vi "Test.vi"() -> ()   [LabVIEW 2009]
uses:
  LV-BME Interface/BME_DG_TriggerSettings.ctl
  LV-BME Interface/ChnlSettings.ctl
  LV-BME Interface/ChnlWithModulo.ctl
panel:
  out "Array":T1(array[cluster])=[{"Master"=TRUE, "DG_Product"=34, "SlotNumber"=5, "return code"=0}, {"Master"=FALSE, "DG_Product"=33, "SlotNumber"=7, "return code"=0}, {"Master"=FALSE, "DG_Product"=33, "SlotNumber"=9, "return code"=0}, {"Master"=FALSE, "DG_Product"=33, "SlotNumber"=11, "return code"=0}]
  in  "Chnl Settings T, A, B":T2[](array[typedef])=[{" Delay (µs)"=0.0, "TriggerModulo"=1, "On? (false)"=TRUE, "PositiveVoltage?(true)"=TRUE, "50OhmTerminated? "=FALSE, "25OhmOutput?"=FALSE}, {" Delay (µs)"=0.0, "TriggerModulo"=4, "On? (false)"=TRUE, "PositiveVoltage?(true)"=TRUE, "50OhmTerminated? "=FALSE, "25OhmOutput?"=FALSE}, {" Delay (µs)"=0.0, "TriggerModulo"=8, "On? (false)"=TRUE, "PositiveVoltage?(true)"=TRUE, "50OhmTerminated? "=TRUE, "25OhmOutput?"=FALSE}] {"TriggerModulo" min=1 max=1000000; "Delay (µs)" min=0.0 max=100000000.0 format="%.5f"}
  in  "Chnl Settings T, A, B written":T2[](array[typedef])=[{" Delay (µs)"=0.0, "TriggerModulo"=1, "On? (false)"=TRUE, "PositiveVoltage?(true)"=TRUE, "50OhmTerminated? "=FALSE, "25OhmOutput?"=FALSE}, {" Delay (µs)"=0.0, "TriggerModulo"=4, "On? (false)"=TRUE, "PositiveVoltage?(true)"=TRUE, "50OhmTerminated? "=FALSE, "25OhmOutput?"=FALSE}, {" Delay (µs)"=0.0, "TriggerModulo"=8, "On? (false)"=TRUE, "PositiveVoltage?(true)"=TRUE, "50OhmTerminated? "=TRUE, "25OhmOutput?"=FALSE}] {"TriggerModulo" min=1 max=1000000; "Delay (µs)" min=0.0 max=100000000.0 format="%.5f"}
  out "Update chnl errors":errorcluster[](array[cluster])
  in  "update chnl settings":bool=TRUE
  out "counters remain":u32[](array[numeric])=[1, 2, 6]
  out "activate":i32[](array[numeric])
  in  "Activate":bool=TRUE
  out "Chnl States":i32[][](array[numeric])
  in  "ReadStatus":bool=TRUE
  in  "stop 2":bool=TRUE
  in  "stop":bool=TRUE
  out "errori init":i32[](array[numeric])
  out "errori set trigger":i32[](array[numeric])=[0, -1, -1, -1]
  out "errori set clock":i32[](array[numeric])=[0, -1, -1, -1]
  in  "ChnM B":T3={" Delay (µs)"=1000.0, "On? (false)"=TRUE, "PositiveVoltage?"=TRUE, "50OhmTerminated? "=TRUE, "25OhmOutput?"=FALSE} {"Delay (µs)" min=0.0 max=100000000.0 format="%.5f"}
  in  "ChnM A":T3={" Delay (µs)"=0.0, "On? (false)"=TRUE, "PositiveVoltage?"=TRUE, "50OhmTerminated? "=FALSE, "25OhmOutput?"=FALSE} {"Delay (µs)" min=0.0 max=100000000.0 format="%.5f"}
  in  "ChnM T":T3={" Delay (µs)"=0.0, "On? (false)"=TRUE, "PositiveVoltage?"=TRUE, "50OhmTerminated? "=FALSE, "25OhmOutput?"=FALSE} {"Delay (µs)" min=0.0 max=100000000.0 format="%.5f"}
  in  "Trigger Settings":T4={"InputTerminated?"=FALSE, "InternalClockPeriode(µs)"=1000000.0, "TriggerLevel"=1.25, "PresetValue"=0, "DivideBy"=1, "Clock Source"=1, "Gate Divider"=1, "PositiveGate?"=TRUE, "InternalTrigger?"=TRUE, "InternalArm?"=FALSE, "SWTrigger?"=FALSE, "RisingEdge?"=FALSE, "StopOnPreset?"=FALSE, "ResetWhenDone?"=TRUE, "TriggerEnabled?"=TRUE} {"Gate Divider" min=1 max=1000000; "Clock Source" items=["Internal Oscillator"=1, "External Trigger"=2, "Trigger & Oscillator"=3]}
  out "NumberOfCards":i32=4
  out "error out":errorcluster
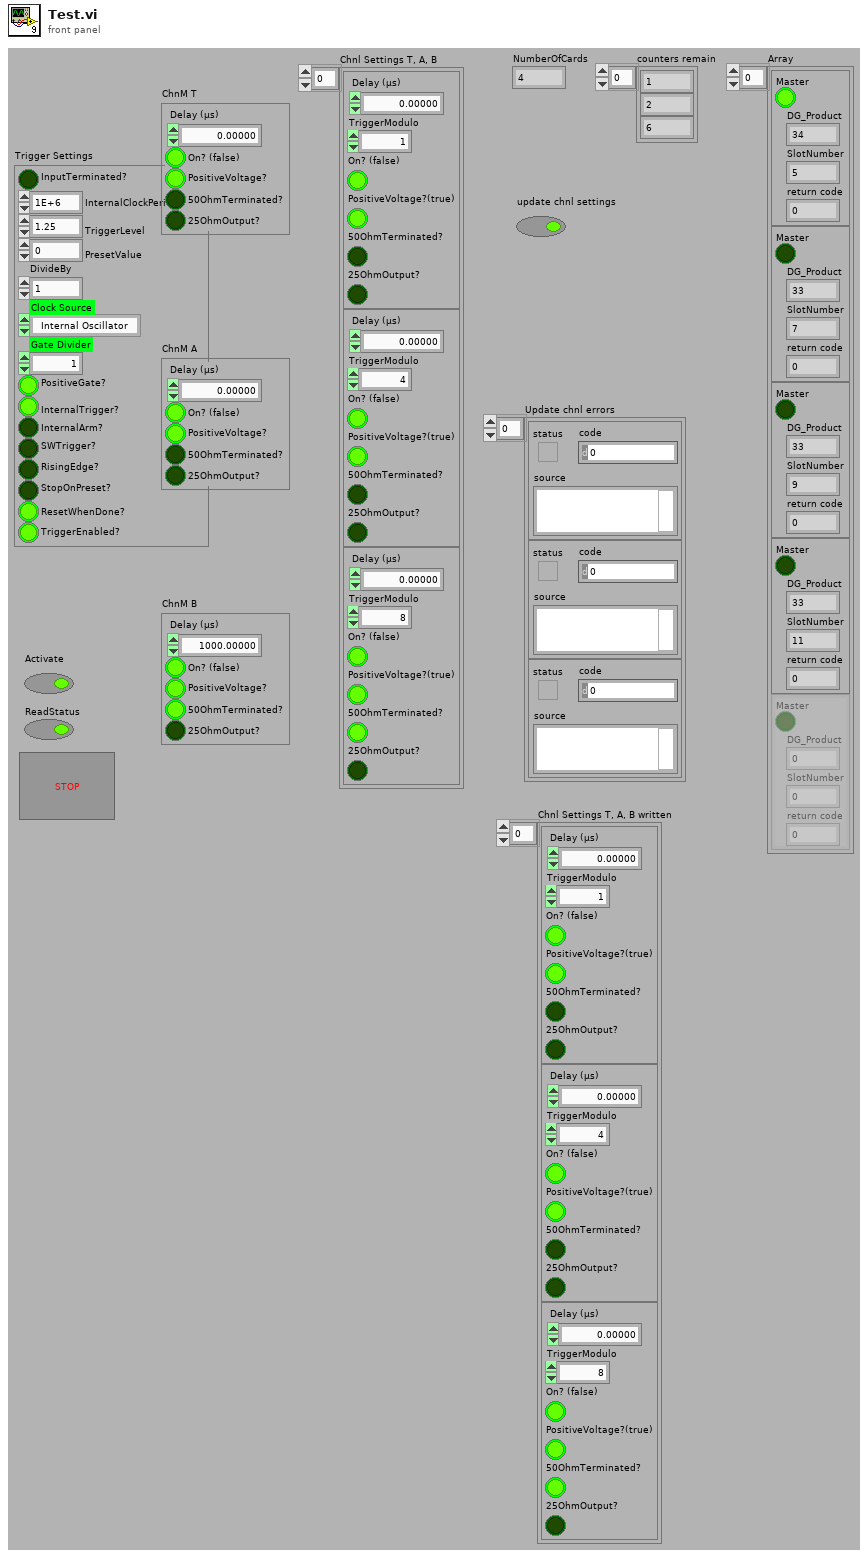
[diagram p1: front panel]
types:
  T1 = cluster{"Master":bool, "DG_Product":i32, "SlotNumber":i32, "return code":i32}[]
  T2 = typedef "ChnlWithModulo.ctl" = cluster{" Delay (µs)":dbl, "TriggerModulo":u32, "On? (false)":bool, "PositiveVoltage?(true)":bool, "50OhmTerminated? ":bool, "25OhmOutput?":bool}
  T3 = typedef "ChnlSettings.ctl" = cluster{" Delay (µs)":dbl, "On? (false)":bool, "PositiveVoltage?":bool, "50OhmTerminated? ":bool, "25OhmOutput?":bool}
  T4 = typedef "BME_DG_TriggerSettings.ctl" = cluster{"InputTerminated?":bool, "InternalClockPeriode(µs)":dbl, "TriggerLevel":dbl, "PresetValue":i32, "DivideBy":i32, "Clock Source":u32, "Gate Divider":i32, "PositiveGate?":bool, "InternalTrigger?":bool, "InternalArm?":bool, "SWTrigger?":bool, "RisingEdge?":bool, "StopOnPreset?":bool, "ResetWhenDone?":bool, "TriggerEnabled?":bool}
  T5 = cluster{"Master":bool, "DG_Product":i32, "SlotNumber":i32, "return code":i32}
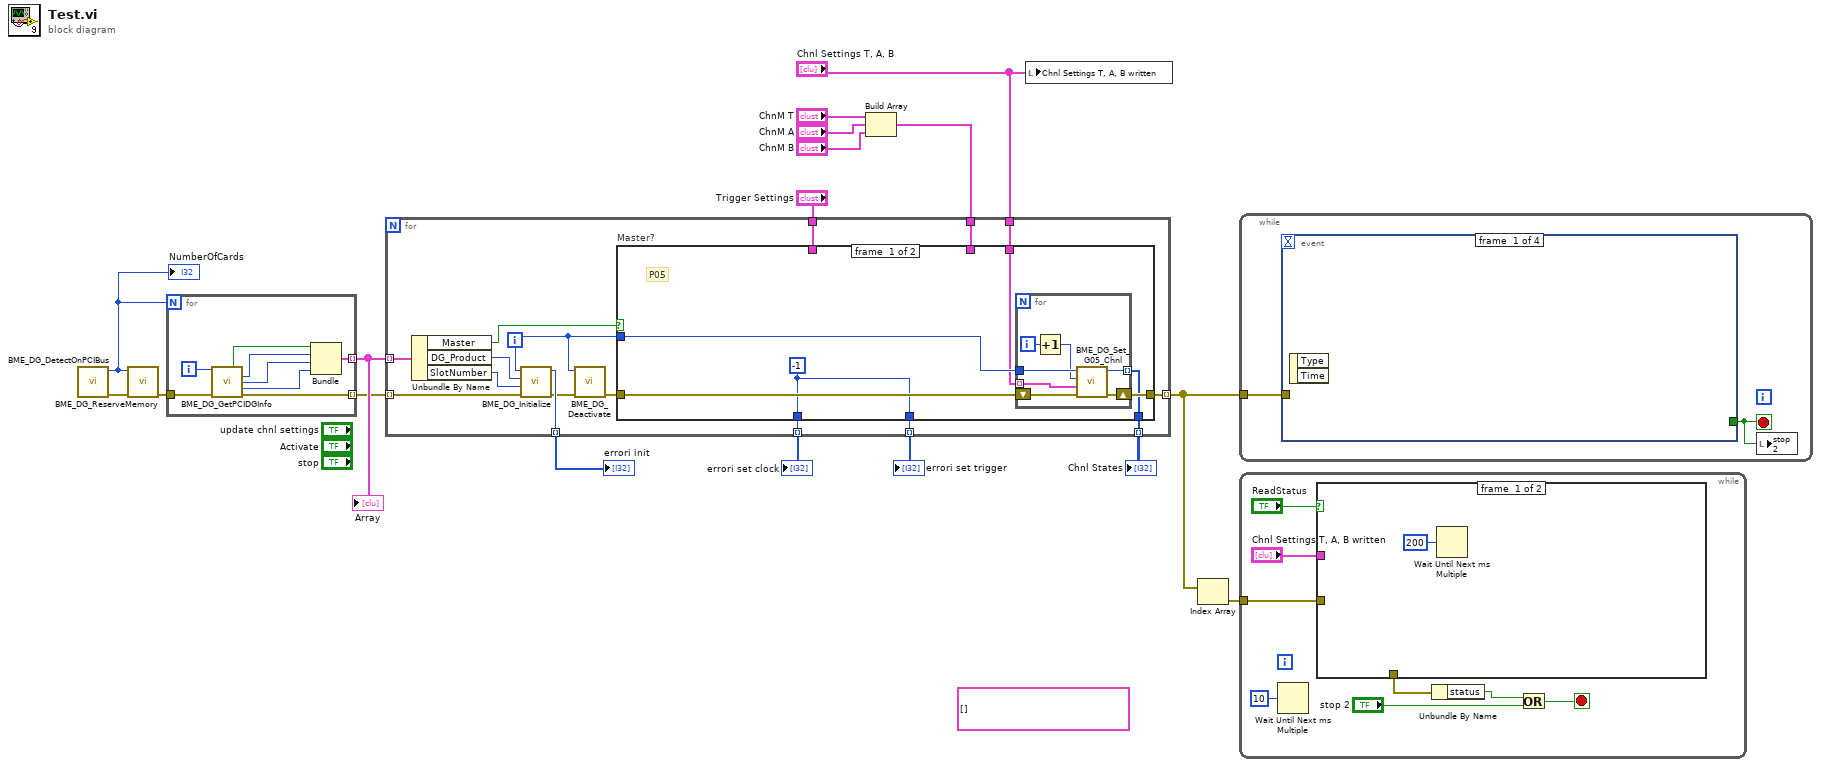
[diagram p0: block diagram]
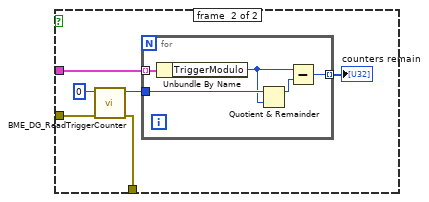
[diagram p2: hidden frame]
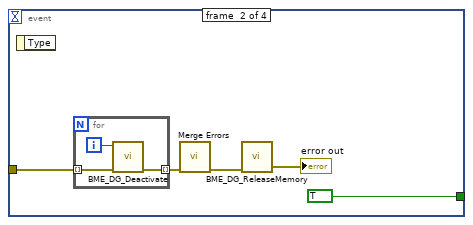
[diagram p3: hidden frame]
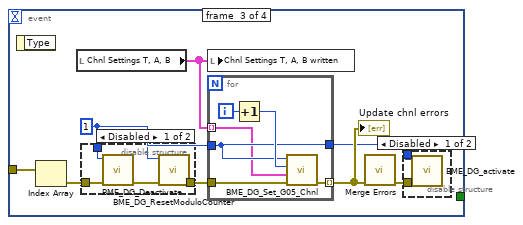
[diagram p4: hidden frame]
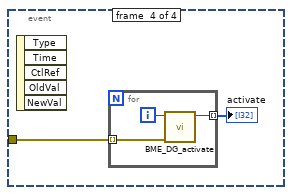
[diagram p7: hidden frame]
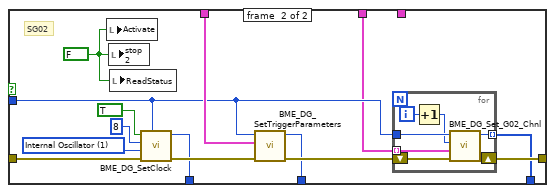
[diagram p8: hidden frame]
diagram:
  (unwired) cluster{"Time":string, "state":i32}[] []
  n1 = call "BME_DG_DetectOnPCIBus.vi"() -> ("error out"=w17:errorcluster, "NumberOfCards"=w3:i32)  [unwired: 9 in, 1 out]
  "NumberOfCards" <- w3
  n2 = call "BME_DG_ReserveMemory.vi"("error in (no error)"=w17, "Number of Cards"=w3) -> ("error out"=w16:errorcluster)  [unwired: 8 in, 1 out]
  n3 = for {
    N: w3 -> [_]
    tunnel: [w23] -> w14 mode=indexing
    tunnel: [w18] -> w15 mode=indexing
    tunnel: w16 -> [w24]
    i -> [w25]
    n4 = call "BME_DG_GetPCIDGInfo.vi"("DG_Number in"=w25, "error in (no error)"=w24) -> ("Master"=w22:bool, "DG_Product"=w21:i32, "SlotNumber"=w20:i32, "return code"=w19:i32, "error out"=w23:errorcluster)  [unwired: 8 in, 1 out]
    n5 = Bundle("Master"=w22, "DG_Product"=w21, "SlotNumber"=w20, "return code"=w19) -> (w18:T5)  [unwired: 1 in]
  }
  "Array" <- w15
  n6 = Build Array("ChnM T", "ChnM A", "ChnM B") -> (w9:T3[])
  n7 = for {
    tunnel: w15 -> [w41] mode=indexing
    tunnel: w14 -> [w40] mode=indexing
    tunnel: [w39] -> w6 mode=indexing
    tunnel: [w37] -> w5 mode=indexing
    tunnel: "Trigger Settings" -> [w36]
    tunnel: w9 -> [w35]
    tunnel: "Chnl Settings T, A, B" -> [w34]
    tunnel: [w33] -> w8 mode=indexing
    tunnel: [w32] -> w7 mode=indexing
    tunnel: [w31] -> w4 mode=indexing
    i -> [w28]
    n8 = Unbundle By Name(w41) -> ("Master"=w38:bool, "DG_Product"=w27:i32, "SlotNumber"=w26:i32)
    n9 = call "BME_DG_Initialize.vi"("error in (no error)"=w40, "Slot Number"=w26, "DG_Product"=w27, "DG_Number"=w28) -> ("error out"=w30:errorcluster, "return code"=w39:i32)  [unwired: 5 in]
    n10 = call "BME_DG_Deactivate.vi"("error in (no error)"=w30, "DG_Number"=w28) -> ("error out"=w29:errorcluster)  [unwired: 8 in, 1 out]
    n11 = case "Master?" shown="True" w38 {
      tunnel: w29 -> [w47 w68]
      tunnel: w28 -> [w45 w61]
      tunnel: [w46 w62] -> w37
      tunnel: w36 -> [_ w64]
      tunnel: w35 -> [_ w60]
      tunnel: w34 -> [w44 _]
      tunnel: [w43 w59] -> w33
      tunnel: [w43 w58] -> w32
      tunnel: [w42 w57] -> w31
      frame #0 {
        w43 = -1 ("return code")
        # "P05"
        n12 = for {
          tunnel: w45 -> [w54]
          tunnel: w44 -> [w50] mode=indexing
          shift-right: [w52] -> w46
          shift-left: w47 -> [w53]
          tunnel: [w49] -> w42 mode=indexing
          i -> [w51]
          n13 = Increment(x=w51) -> (x+1=w48:i32)
          n14 = call "BME_DG_Set_G05_Chnl.vi"("error in (no error)"=w53, "ChnParameter"=w50, "Channel"=w48, "DG_Number"=w54) -> ("error out"=w52:errorcluster, "return code"=w49:i32)  [unwired: 6 in]
        }
      }
      frame #1 {
        w55 = FALSE ("stop 2")
        w66 = 1 items=["Internal Oscillator"=1, "External Trigger"=2, "Trigger & Oscillator"=3] ("ClockSource")
        # "SG02"
        n15 = local write "Activate"(w55) -> ()
        n16 = local write "stop 2"(w55) -> ()
        n17 = local write "ReadStatus"(w55) -> ()
        n18 = call "BME_DG_SetClock.vi"("DG_NumberM"=w61, "error in (no error)"=w68, "ClockSource"=w66, "DivideBy"=u32 8, "ClockEnable"=TRUE) -> ("error out"=w65:errorcluster, "return code"=w59:i32)  [unwired: 5 in]
        n19 = call "BME_DG_SetTriggerParameters.vi"("error in (no error)"=w65, "Trigger Settings"=w64, "DG_NumberM"=w61) -> ("error out"=w63:errorcluster, "return code"=w58:i32)  [unwired: 7 in]
        n20 = for {
          tunnel: w61 -> [w73]
          tunnel: w60 -> [w71] mode=indexing
          shift-right: [w74] -> w62
          shift-left: w63 -> [w75]
          tunnel: [w70] -> w57 mode=indexing
          i -> [w72]
          n21 = Increment(x=w72) -> (x+1=w69:i32)
          n22 = call "BME_DG_Set_G02_Chnl.vi"("error in (no error)"=w75, "ChnParemater"=w71, "Channel"=w69, "DG_Number"=w73) -> ("error out"=w74:errorcluster, "return code"=w70:i32)  [unwired: 6 in]
        }
      }
    }
  }
  "errori set clock" <- w8
  "errori set trigger" <- w7
  "errori init" <- w6
  "Chnl States" <- w4
  n23 = local write "Chnl Settings T, A, B written"("Chnl Settings T, A, B") -> ()
  n24 = Index Array(array=w5) -> (element=w2:errorcluster)  [unwired: 1 in]
  n25 = while {
    tunnel: w5 -> [w77]
    stop <- w76 stop-if-true
    n26 = event shown="[1] \"stop\": Value Change" {
      selector: _ -> [_ _ _ _]
      dyn-events: _ -> [_ _ _ _]
      timeout: _ -> [_ _ _ _]
      tunnel: [_ TRUE _ _] -> w76
      tunnel: w77 -> [_ w78 w93 w108]
      event #0 {
        n27 = event-data() -> ()  [unwired: 1 in, 2 out]
      }
      event #1 {
        n28 = event-data() -> ()  [unwired: 1 in, 1 out]
        n29 = for {
          tunnel: w78 -> [w85] mode=indexing
          tunnel: [w83] -> w79 mode=indexing
          i -> [w84]
          n30 = call "BME_DG_Deactivate.vi"("error in (no error)"=w85, "DG_Number"=w84) -> ("error out"=w83:errorcluster)  [unwired: 8 in, 1 out]
        }
        n31 = call <vilib>:"Merge Errors.vi"("error array in"=w79) -> ("error out"=w80:errorcluster)  [unwired: 6 in]
        n32 = call "BME_DG_ReleaseMemory.vi"("error in (no error)"=w80) -> ("error out"=→"error out":errorcluster)  [unwired: 9 in, 1 out]
      }
      event #2 {
        w87 = 1 ("DG_Number")
        n33 = event-data() -> ()  [unwired: 1 in, 1 out]
        n34 = Index Array(array=w93) -> (element=w92:errorcluster)  [unwired: 1 in]
        n35 = local read "Chnl Settings T, A, B"() -> (w86:T2[])
        n36 = disable-structure shown="Disabled" {
          disable-tunnel: w92 -> [w99 w100]
          disable-tunnel: [w97 w100] -> w88
          disable-tunnel: w87 -> [w96 _]
          frame #0 {
            n37 = call "BME_DG_Deactivate.vi"("error in (no error)"=w99, "DG_Number"=w96) -> ("error out"=w98:errorcluster)  [unwired: 8 in, 1 out]
            n38 = call "BME_DG_ResetModuloCounter.vi"("error in (no error)"=w98, "DG_Number"=w96) -> ("error out"=w97:errorcluster)  [unwired: 8 in, 1 out]
          }
          frame #1 {
          }
        }
        n39 = local write "Chnl Settings T, A, B written"(w86) -> ()
        n40 = for {
          tunnel: w86 -> [w101] mode=indexing
          tunnel: w88 -> [w104]
          tunnel: [w103] -> w91 mode=indexing
          tunnel: w87 -> [w102]
          tunnel: [w102] -> w89
          i -> [w106]
          n41 = Increment(x=w106) -> (x+1=w105:i32)
          n42 = call "BME_DG_Set_G05_Chnl.vi"("error in (no error)"=w104, "ChnParameter"=w101, "Channel"=w105, "DG_Number"=w102) -> ("error out"=w103:errorcluster)  [unwired: 6 in, 1 out]
        }
        "Update chnl errors" <- w91
        n43 = call <vilib>:"Merge Errors.vi"("error array in"=w91) -> ("error out"=w90:errorcluster)  [unwired: 6 in]
        n44 = disable-structure shown="Disabled" {
          disable-tunnel: w90 -> [w95 _]
          disable-tunnel: w89 -> [w94 _]
          frame #0 {
            n45 = call "BME_DG_activate.vi"("error in (no error)"=w95, "DG_Number"=w94) -> ()  [unwired: 8 in, 2 out]
          }
          frame #1 {
          }
        }
      }
      event #3 {
        n46 = event-data() -> ()  [unwired: 1 in, 5 out]
        n47 = for {
          tunnel: w108 -> [w111] mode=indexing
          tunnel: [w109] -> w107 mode=indexing
          i -> [w110]
          n48 = call "BME_DG_activate.vi"("error in (no error)"=w111, "DG_Number"=w110) -> ("return code"=w109:i32)  [unwired: 8 in, 1 out]
        }
        "activate" <- w107
      }
    }
    n49 = local write "stop 2"(w76) -> ()
  }
  n50 = while {
    tunnel: w2 -> [w119]
    stop <- w116 stop-if-true
    n51 = Wait Until Next ms Multiple(millisecond multiple=u32 10) -> ()  [unwired: 1 out]
    n52 = case shown="True" "ReadStatus" {
      tunnel: w119 -> [_ w121]
      tunnel: [_ w126] -> w114
      tunnel: "Chnl Settings T, A, B written" -> [_ w125]
      frame #0 {
        n53 = Wait Until Next ms Multiple(millisecond multiple=u32 200) -> ()  [unwired: 1 out]
      }
      frame #1 {
        n54 = call "BME_DG_ReadTriggerCounter.vi"("error in (no error)"=w121, "DG_Number"=0) -> ("error out"=w126:errorcluster, "return value"=w122:i32)  [unwired: 8 in]
        n55 = for {
          tunnel: w125 -> [w131] mode=indexing
          tunnel: w122 -> [w130]
          tunnel: [w128] -> w124 mode=indexing
          n56 = Unbundle By Name(w131) -> ("TriggerModulo"=w127:u32)
          n57 = Quotient & Remainder(x=w130, y=w127) -> (x-y*floor(x/y)=w129:u32)  [unwired: 1 out]
          n58 = Subtract(x=w127, y=w129) -> (x-y=w128:u32)
        }
        "counters remain" <- w124
      }
    }
    n59 = Unbundle By Name(w114) -> ("status"=w115:bool)
    n60 = Or(x=w115, y="stop 2") -> (x .or. y?=w116:bool)
  }
